vi "Run Filter.vi"(8 "error in (no error)":errorcluster, 10 "resource entries in":T1[](array[typedef]) {"FPGA CD Ref" format="%.0x"; "reserver" format="%.0x"}, 11 "XOR Filter in":refnum<class "XOR Filter.lvclass">) -> (0 "error out":errorcluster, 2 "resource entries out":T1[](array[typedef]) {"FPGA CD Ref" format="%.0x"; "reserver" format="%.0x"})   [LabVIEW 2016, in "FPGA Resource Manager.lvlib" / "XOR Filter.lvclass"]
uses:
  XOR Filter.lvclass
  Server/resource info.ctl
  <vilib>/NI Veristand/Custom Device API/Custom Device Item Ref.ctl
  XOR Filter.lvclass/XOR Filter.ctl
  Filter Parent/Filter.lvclass
  NOT Filter/NOT Filter.lvclass
  And Filter/AND Filter.lvclass
  OR Filter/OR Filter.lvclass
  <vilib>/NI VeriStand/Custom Device API/Custom Device API.lvlib
  FPGA Resource Manager.lvlib
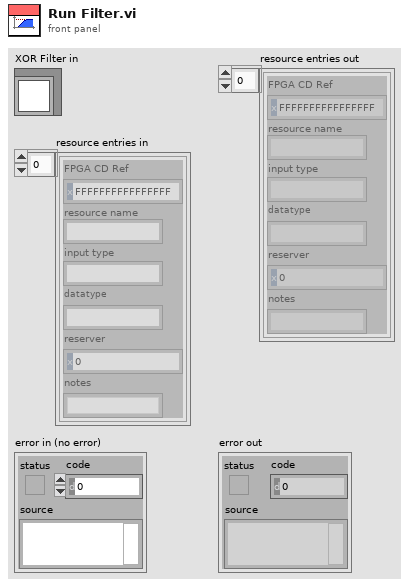
[diagram p1: front panel]
types:
  T1 = typedef "FPGA Resource Manager.lvlib/resource info.ctl" = cluster{"FPGA CD Ref":T2, "resource name":string, "input type":string, "datatype":string, "reserver":T2, "notes":string}
  T2 = typedef "Custom Device API.lvlib/Custom Device Item Ref.ctl" = u64
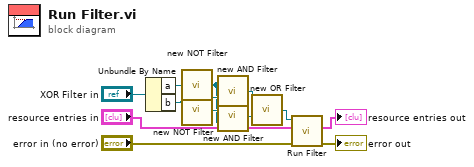
[diagram p0: block diagram]
diagram:
  n1 = Unbundle By Name("XOR Filter in") -> ("a"=w11:refnum<class "Filter.lvclass">, "b"=w10:refnum<class "Filter.lvclass">)
  n2 = call "new NOT Filter.vi"("a"=w11) -> ("not a"=w8:refnum<class "Filter.lvclass">)  [unwired: 14 in]
  n3 = call "new NOT Filter.vi"("a"=w10) -> ("not a"=w9:refnum<class "Filter.lvclass">)  [unwired: 14 in]
  n4 = call "new AND Filter.vi"("a"=w8, "b"=w10) -> ("a and b"=w7:refnum<class "Filter.lvclass">)  [unwired: 13 in]
  n5 = call "new AND Filter.vi"("a"=w9, "b"=w8) -> ("a and b"=w6:refnum<class "Filter.lvclass">)  [unwired: 13 in]
  n6 = call "new OR Filter.vi"("a"=w7, "b"=w6) -> ("a or b"=w5:refnum<class "Filter.lvclass">)  [unwired: 13 in]
  n7 = call-dynamic "Run Filter.vi"("error in (no error)"="error in (no error)", "resource entries in"="resource entries in", "Filter in"=w5) -> ("error out"=→"error out":errorcluster, "resource entries out"=→"resource entries out":T1[])  [unwired: 7 in]
